vi "Main.vi"(6 "DVR API Suffix":string=" API", 8 "error in (no error)":errorcluster, 9 "DVR API Directory Path":path, 10 "Class Method Directory":path, 11 "Class Path":path) -> (0 "error out":errorcluster)   [LabVIEW 2016, in "SLL Class DVR API Generator.lvlib"]
uses:
  SLL Class DVR API Generator.lvlib
panel:
  out "DVR API Count":i32
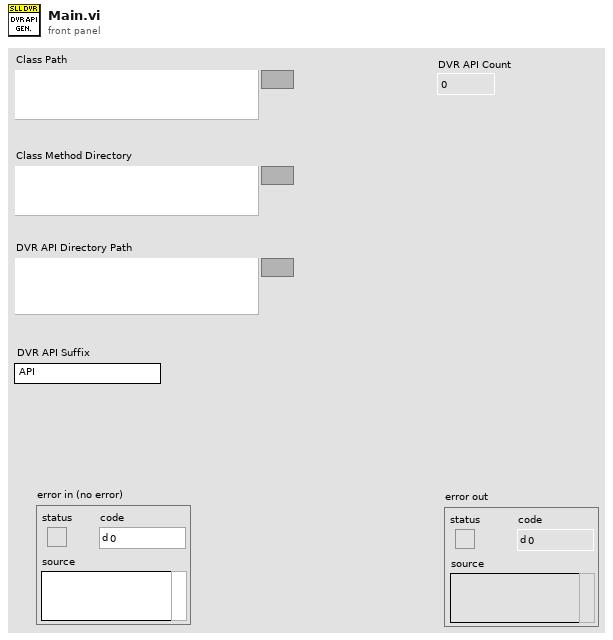
[diagram p1: front panel]
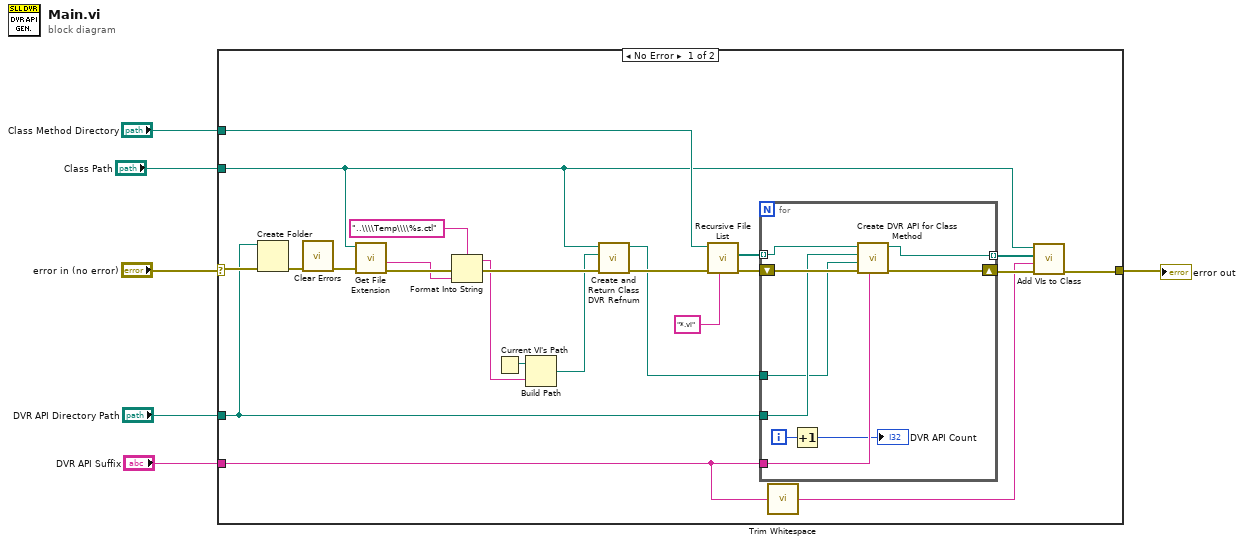
[diagram p0: block diagram]
diagram:
  n1 = case shown="No Error" "error in (no error)" {
    selector: "error in (no error)" -> [w10 w39]
    tunnel: [w15 w39] -> w5
    tunnel: "Class Path" -> [w14 _]
    tunnel: "DVR API Suffix" -> [w13 _]
    tunnel: "Class Method Directory" -> [w19 _]
    tunnel: "DVR API Directory Path" -> [w8 _]
    frame No Error {
      n2 = Create Folder(path (use dialog)=w8, error in=w10) -> (error out=w9:errorcluster)  [unwired: 1 in, 2 out]
      n3 = call <vilib>:"Clear Errors.vi"("error in (no error)"=w9) -> ("error out"=w7:errorcluster)  [unwired: 5 in, 1 out]
      n4 = call <vilib>:"Get File Extension.vi"("error in (no error)"=w7, "file"=w14) -> ("error out"=w25:errorcluster, "filename without extension"=w24:string)  [unwired: 5 in, 3 out]
      n5 = Format Into String(format string="..\\\\Temp\\\\%s.ctl", error in=w25, w24) -> (resulting string=w27:string, error out=w29:errorcluster)  [unwired: 1 in]
      n6 = Current VI's Path() -> (path=w26:path)
      n7 = Build Path(base path=w26, name or relative path=w27) -> (appended path=w22:path)
      n8 = call "Create and Return Class DVR Refnum.vi"("error in (no error)"=w29, "Path to Save DVR Class Control"=w22, "Class Path"=w14) -> ("error out"=w23:errorcluster, "DVR Class Control Path Out"=w18:path)  [unwired: 7 in]
      n9 = call <vilib>:"Recursive File List.vi"("pattern"="*.vi", "error in (no error)"=w23, "Folder Path"=w19) -> ("error out"=w21:errorcluster, "All Files in Dir"=w17:path[])  [unwired: 4 in, 3 out]
      n10 = for {
        tunnel: w13 -> [w33]
        tunnel: w8 -> [w36]
        tunnel: w18 -> [w35]
        shift-right: [w38] -> w16
        shift-left: w21 -> [w37]
        tunnel: w17 -> [w34] mode=indexing
        tunnel: [w32] -> w11 mode=indexing
        i -> [w31]
        n11 = Increment(x=w31) -> (x+1=→"DVR API Count":i32)
        n12 = call "Create DVR API for Class Method.vi"("DVR API Suffix"=w33, "error in (no error)"=w37, "Class DVR Control File Path"=w35, "DVR API Directory Path"=w36, "Class Method Path"=w34) -> ("error out"=w38:errorcluster, "DVR VI Path"=w32:path)  [unwired: 5 in]
      }
      n13 = call <vilib>:"Trim Whitespace.vi"("string"=w13) -> ("trimmed string"=w12:string)  [unwired: 1 in]
      n14 = call "Add VIs to Class.vi"("error in (no error)"=w16, "Folder Name"=w12, "DVR VI Paths[]"=w11, "Class Path"=w14) -> ("error out"=w15:errorcluster)  [unwired: 7 in]
    }
    frame Error {
    }
  }
  "error out" <- w5
